vi "Test Sequence.vi"(0 "FeedBack Channel":string[](array[string])=["fgdgfvcbc", "vnfhgjkn", "21354682"], 1 "Test Name":string, 2 "Steps":T1(array[cluster]), 3 "Load":refnum<vi>, 4 "Lvdt":refnum<vi>) -> (6 "Emergency":bool, 7 "Out":i32, 8 "Condition":bool)   [LabVIEW 2020]
uses:
  Galobal variable_TI.vi
  Project Setup/Globle Variable/GR_Servo.vi
panel:
  out "Wait/Poll (ms)":u32
  out "Channels (Out)":i32[](array[numeric])
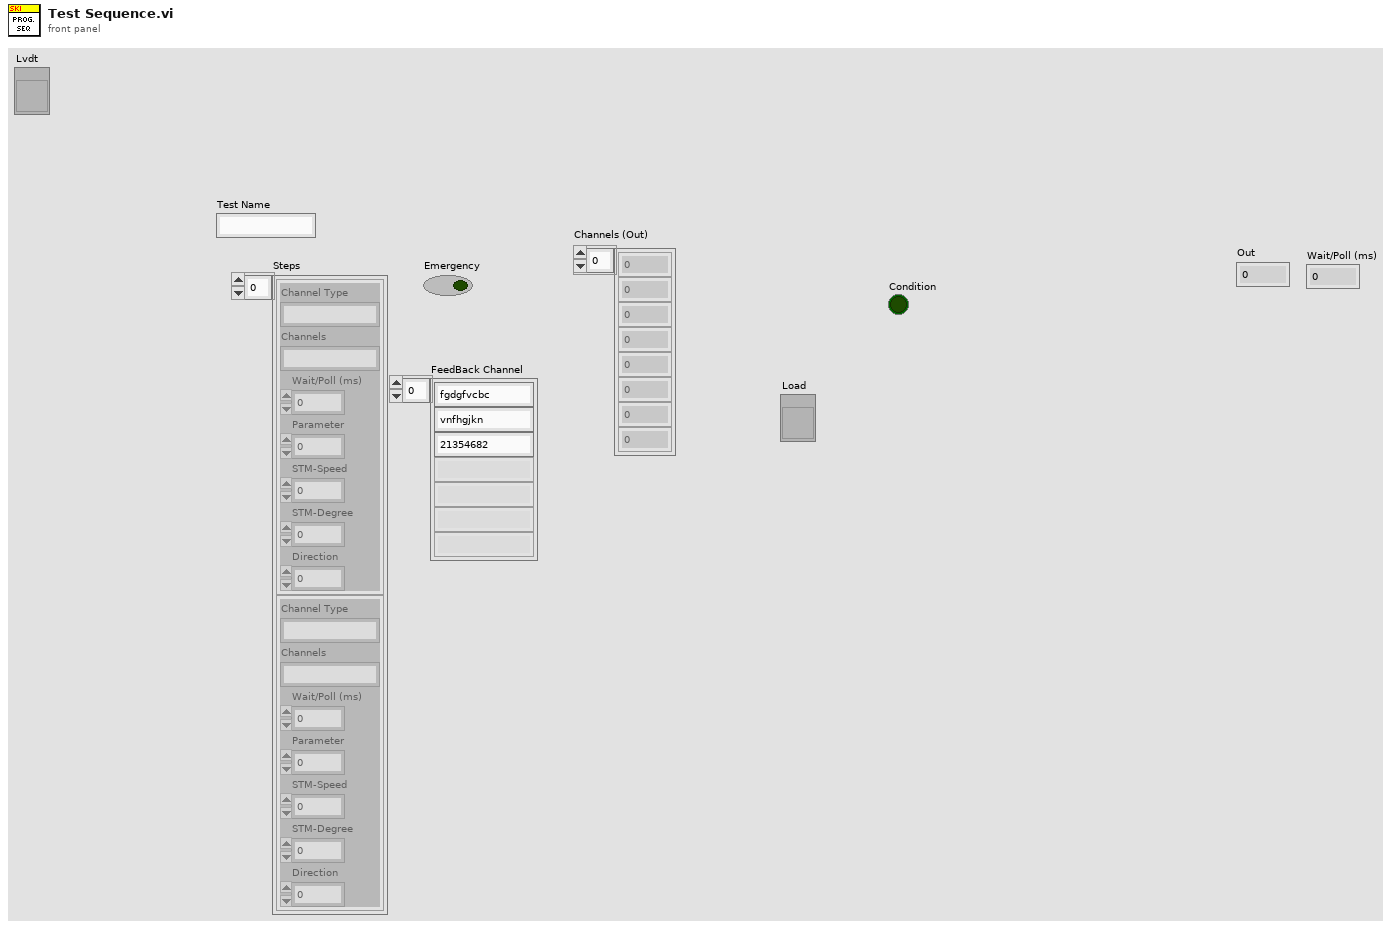
[diagram p1: front panel]
types:
  T1 = cluster{"Channel Type":string, "Channels":string, "Wait/Poll (ms)":u32, "Parameter":u8, "STM-Speed":i32, "STM-Degree":u32, "Direction":u8}[]
  T2 = cluster{"Emergency_1":bool, "Reset_2":bool, "Air Pressure_4":bool, "Safety Sensor_5":bool, "Safety Sensor_6":bool, "Barcode Rev rs_24":bool, "Clamp fwd rs_21":bool, "Servo Fault":bool, "Home _3":bool}
  T3 = cluster{"Start":bool, "Emergency ":bool, "Reset":bool, "Home":bool, "Safety":bool}
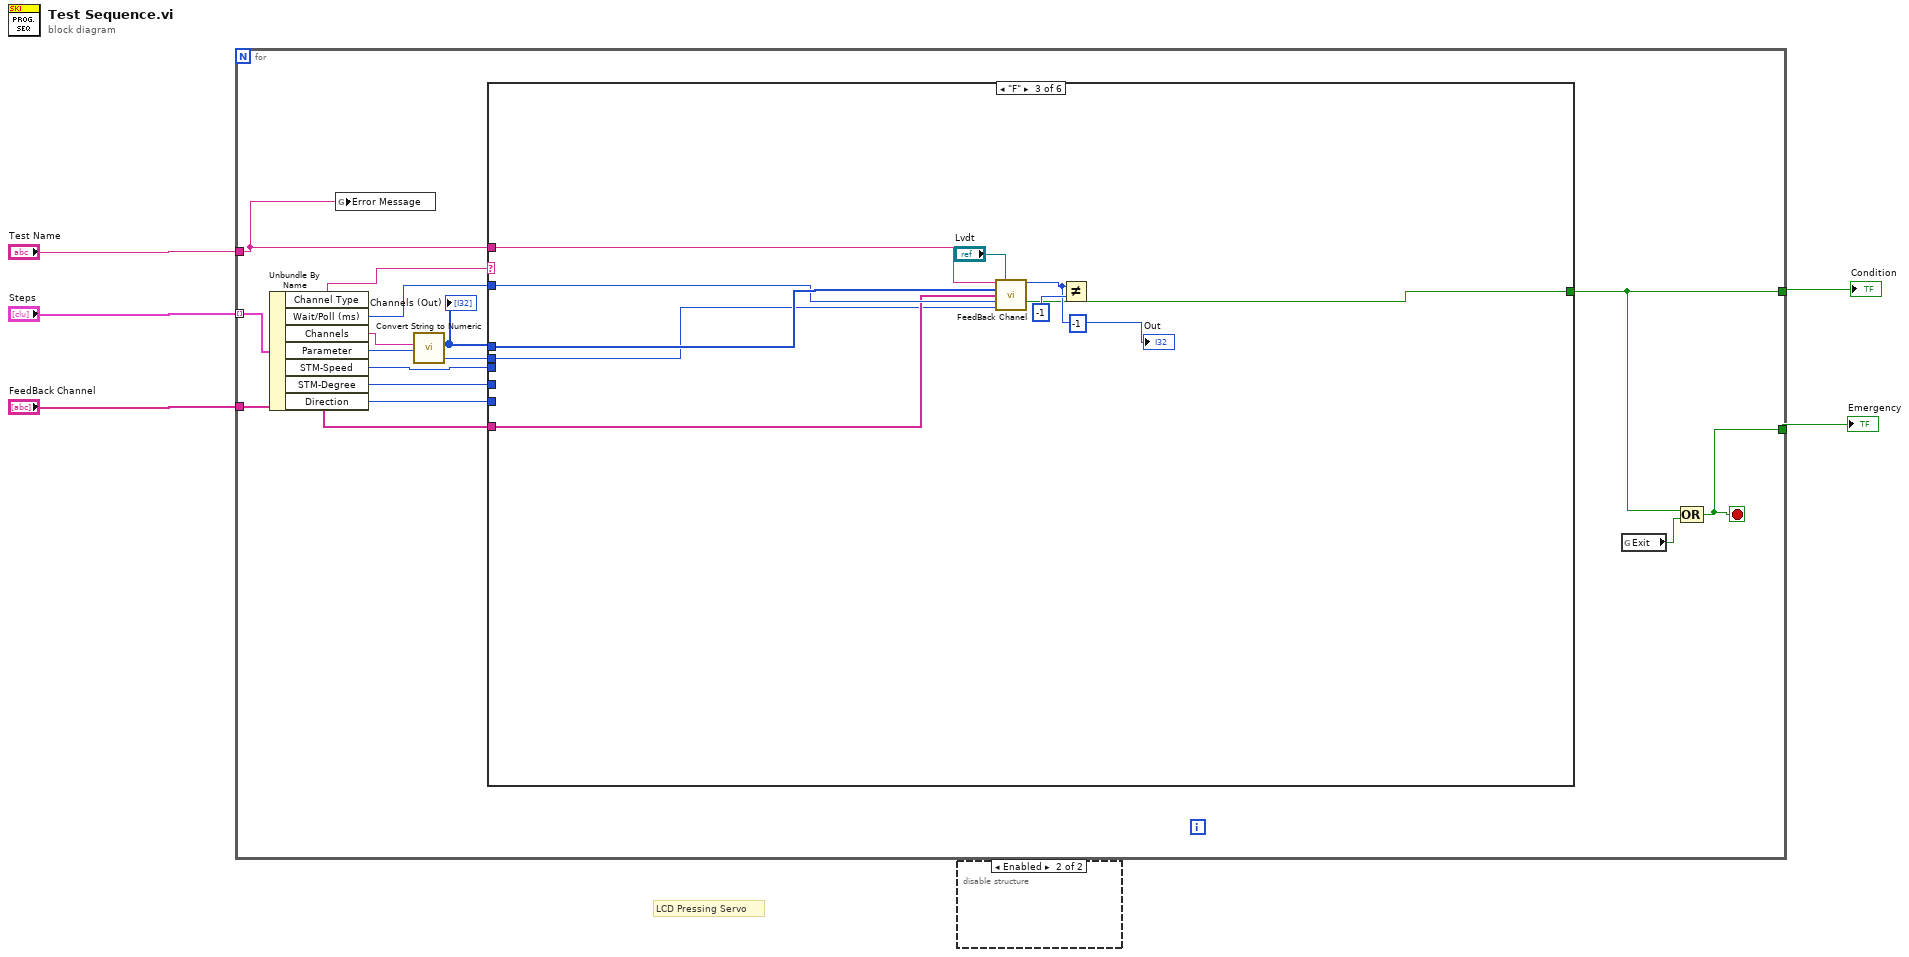
[diagram p0: block diagram]
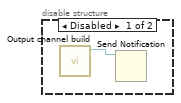
[diagram p2: hidden frame]
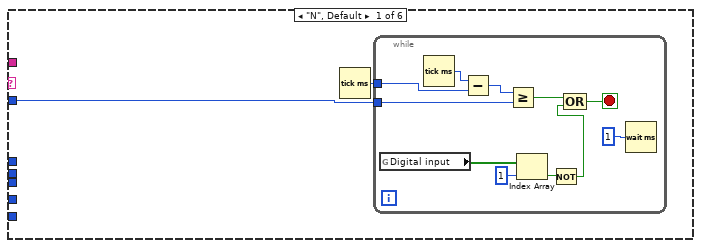
[diagram p3: hidden frame]
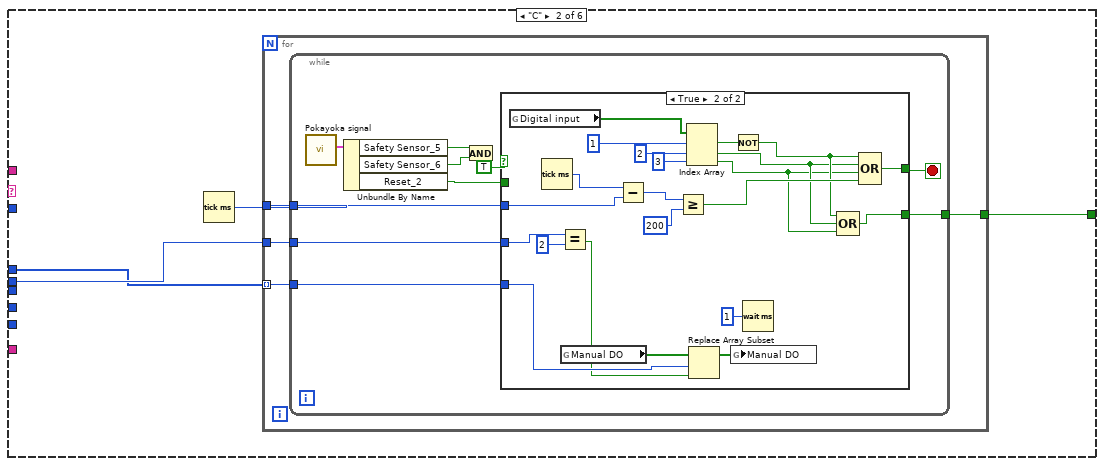
[diagram p4: hidden frame]
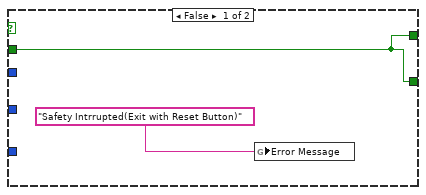
[diagram p5: hidden frame]
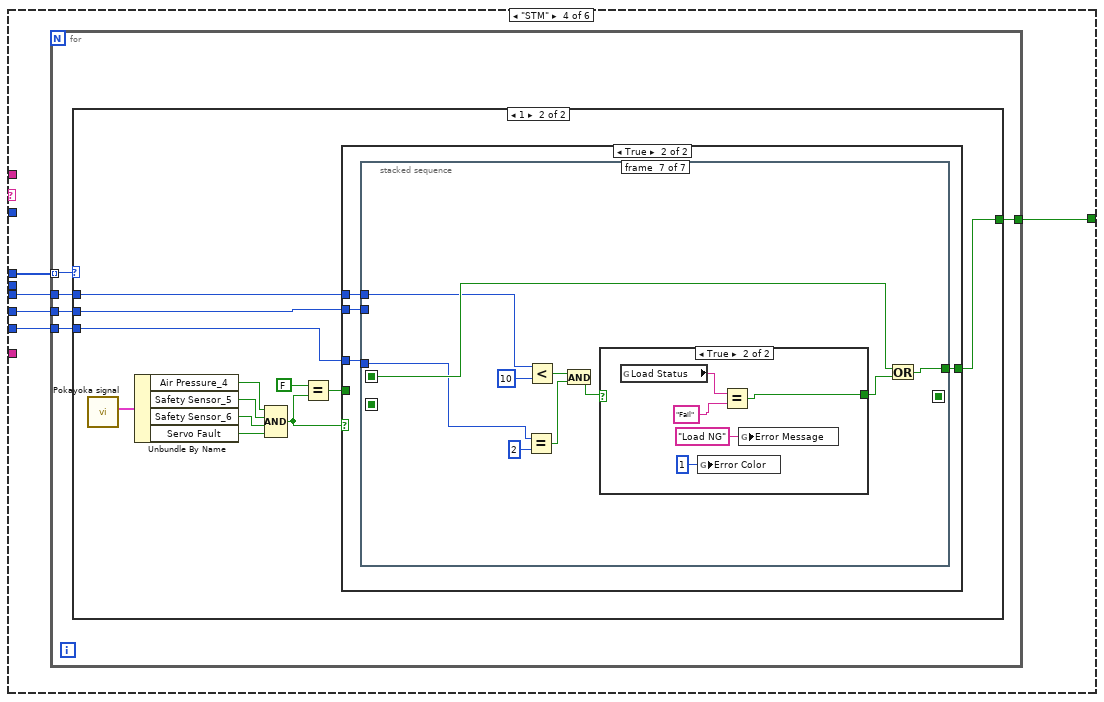
[diagram p6: hidden frame]
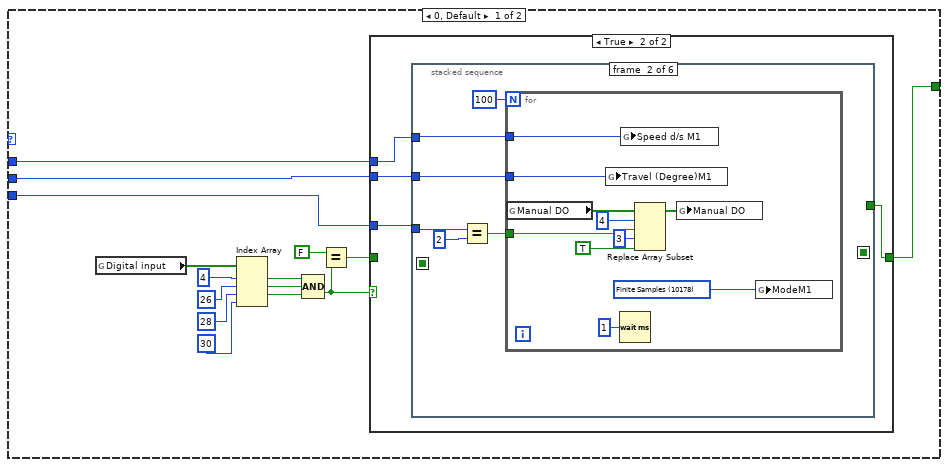
[diagram p7: hidden frame]
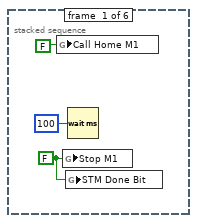
[diagram p9: hidden frame]
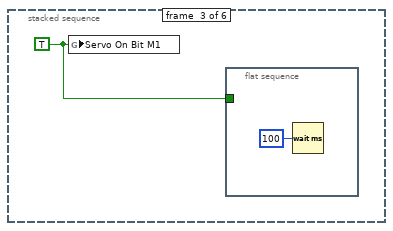
[diagram p10: hidden frame]
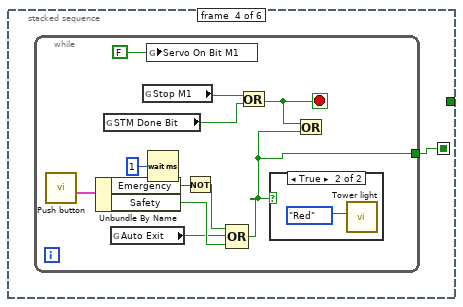
[diagram p11: hidden frame]
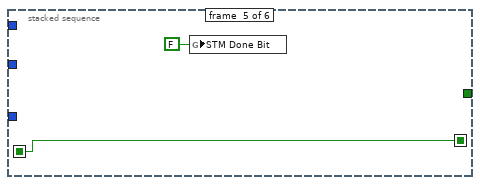
[diagram p13: hidden frame]
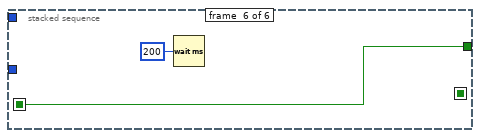
[diagram p14: hidden frame]
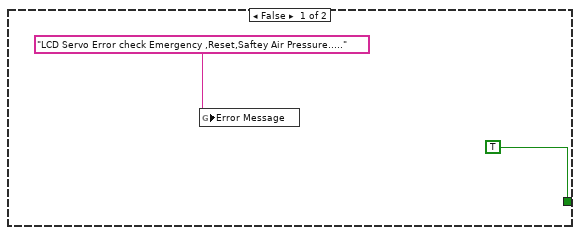
[diagram p15: hidden frame]
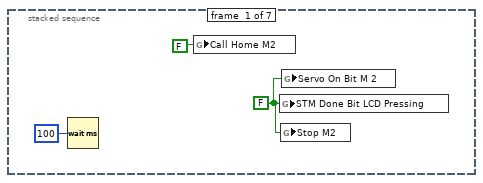
[diagram p16: hidden frame]
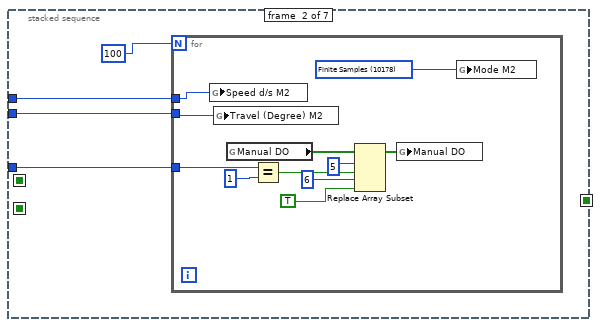
[diagram p17: hidden frame]
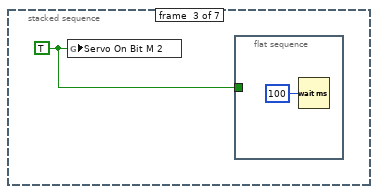
[diagram p18: hidden frame]
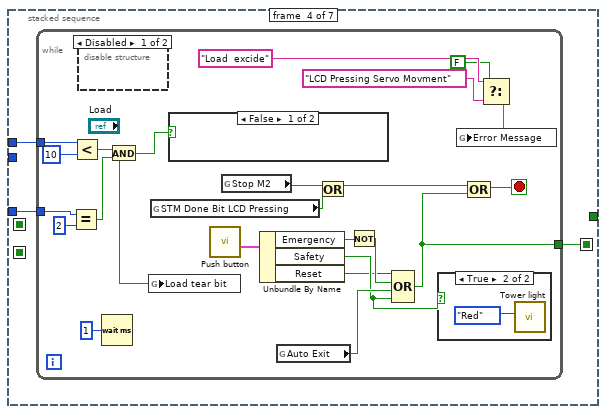
[diagram p19: hidden frame]
diagram:
  # "LCD Pressing Servo"
  n1 = for {
    tunnel: "Steps" -> [w19] mode=indexing
    tunnel: [w7] -> w5
    tunnel: "Test Name" -> [w6]
    tunnel: "FeedBack Channel" -> [w14]
    tunnel: [w12] -> w1
    stop <- w7 stop-if-true
    n2 = Unbundle By Name(w19) -> ("Channel Type"=w18:string, "Wait/Poll (ms)"=w17:u32, "Channels"=w16:string, "Parameter"=w8:u8, "STM-Speed"=w10:i32, "STM-Degree"=w9:u32, "Direction"=w11:u8)
    n3 = global write "GR_Servo.vi" "Error Message"(w6) -> ()
    n4 = call "Convert String to Numeric.vi"("Channels (A:B:C:D...) (In)"=w16) -> ("Channels (Out)"=w15:i32[])  [unwired: 9 in, 1 out]
    "Channels (Out)" <- w15
    n5 = case shown="\"F\"" w18 {
      tunnel: w17 -> [w20 _ w82 _ _ w277]
      tunnel: w15 -> [_ w34 w83 w88 w245 _]
      tunnel: w11 -> [_ _ _ w87 _ _]
      tunnel: w6 -> [_ _ w81 _ _ _]
      tunnel: w14 -> [_ _ w80 _ _ _]
      tunnel: [_ w33 w76 w84 w243 w273] -> w12
      tunnel: w10 -> [_ _ _ w86 _ _]
      tunnel: w9 -> [_ _ _ w85 _ _]
      tunnel: w8 -> [_ w36 w77 _ w244 w280]
      frame "N", Default {
        n6 = Tick Count (ms)() -> (millisecond timer value=w21:u32)
        n7 = while {
          tunnel: w21 -> [w31]
          tunnel: w20 -> [w26]
          stop <- w27 stop-if-true
          n8 = global read "Galobal variable_TI.vi" "Digital input"() -> (w25:bool[])
          n9 = Tick Count (ms)() -> (millisecond timer value=w32:u32)
          n10 = Subtract(x=w32, y=w31) -> (x-y=w30:u32)
          n11 = Greater Or Equal?(x=w30, y=w26) -> (x >= y?=w28:bool)
          n12 = Index Array(array=w25, index=1) -> (element=w23:bool)
          n13 = Not(x=w23) -> (.not. x?=w22:bool)
          n14 = Compound Arithmetic op=OR(w28, w22) -> (w27:bool)
          n15 = Wait (ms)(milliseconds to wait=u32 1) -> ()  [unwired: 1 out]
        }
      }
      frame "C" {
        n16 = Tick Count (ms)() -> (millisecond timer value=w35:u32)
        n17 = for {
          tunnel: w34 -> [w39] mode=indexing
          tunnel: w36 -> [w40]
          tunnel: w35 -> [w38]
          tunnel: [w37] -> w33
          n18 = while {
            tunnel: w40 -> [w50]
            tunnel: w39 -> [w49]
            tunnel: w38 -> [w48]
            tunnel: [w42] -> w37
            stop <- w43 stop-if-true
            n19 = call "Pokayoka signal.vi"() -> ("output cluster"=w47:T2)  [unwired: 10 in, 1 out]
            n20 = Unbundle By Name(w47) -> ("Safety Sensor_5"=w46:bool, "Safety Sensor_6"=w45:bool, "Reset_2"=w44:bool)
            n21 = And(x=w46, y=w45) -> ()  [unwired: 1 out]
            n22 = case shown="True" TRUE {
              tunnel: w50 -> [_ w74]
              tunnel: w49 -> [_ w73]
              tunnel: w48 -> [_ w72]
              tunnel: [w51 w71] -> w43
              tunnel: w44 -> [w51 _]
              tunnel: [w51 w53] -> w42
              frame False {
                n23 = global write "GR_Servo.vi" "Error Message"("Safety Intrrupted(Exit with Reset Button)") -> ()
              }
              frame True {
                n24 = global read "Galobal variable_TI.vi" "Digital input"() -> (w61:bool[])
                n25 = Tick Count (ms)() -> (millisecond timer value=w65:u32)
                n26 = Equal?(x=w74, y=u8 2) -> (x = y?=w66:bool)
                n27 = global read "Galobal variable_TI.vi" "Manual DO"() -> (w67:bool[])
                n28 = Subtract(x=w65, y=w72) -> (x-y=w64:u32)
                n29 = Greater Or Equal?(x=w64, y=u32 200) -> (x >= y?=w62:bool)
                n30 = Index Array(array=w61, index #1=1 ("index"), index #2=2 ("index"), index #3=3 ("index")) -> (element #1=w57:bool, element #2=w55:bool, element #3=w54:bool)
                n31 = Replace Array Subset(array=w67, new element=w66, index=w73) -> (w68:bool[])
                n32 = global write "Galobal variable_TI.vi" "Manual DO"(w68) -> ()
                n33 = Not(x=w57) -> (.not. x?=w56:bool)
                n34 = Wait (ms)(milliseconds to wait=u32 1) -> ()  [unwired: 1 out]
                n35 = Compound Arithmetic op=OR(w56, w55, w54) -> (w53:bool)
                n36 = Compound Arithmetic op=OR(w56, w55, w54, w62) -> (w71:bool)
              }
            }
          }
        }
      }
      frame "F" {
        (unwired) -1 ("Out")
        n37 = call "FeedBack Chanel.vi"("Test Name"=w81, "Lvdt"="Lvdt", "Channels (Int)"=w83, "FeedBack Channel"=w80, "Wait/Poll (ms)"=w82, "Parameter"=w77) -> ("Out"=w78:i32, "Fail"=w76:bool)  [unwired: 5 in, 3 out]
        "Out" <- w78
        n38 = Not Equal?(x=w78, y=-1) -> ()  [unwired: 1 out]
      }
      frame "STM" {
        n39 = for {
          tunnel: w88 -> [w93] mode=indexing
          tunnel: w87 -> [w92]
          tunnel: w86 -> [w91]
          tunnel: w85 -> [w90]
          tunnel: [w89] -> w84
          n40 = case shown="1" w93 {
            tunnel: w92 -> [w106 w159]
            tunnel: w91 -> [w108 w161]
            tunnel: w90 -> [w107 w160]
            tunnel: [w94 w158] -> w89
            frame 0, Default {
              n41 = global read "Galobal variable_TI.vi" "Digital input"() -> (w98:bool[])
              n42 = Index Array(array=w98, index #1=4 ("index"), index #2=26 ("index"), index #3=28 ("index"), index #4=30 ("index")) -> (element #1=w105:bool, element #2=w102:bool, element #3=w103:bool)  [unwired: 1 out]
              n43 = Compound Arithmetic op=AND(w105, w102, w103) -> (w97:bool)
              n44 = Equal?(x=FALSE ("y"), y=w97) -> (x = y?=w95:bool)
              n45 = case shown="True" w97 {
                tunnel: w108 -> [_ w113]
                tunnel: w107 -> [_ w112]
                tunnel: w106 -> [_ w111]
                tunnel: [w109 w110] -> w94
                tunnel: w95 -> [w109 _]
                frame False {
                }
                frame True {
                  n46 = stacked-sequence {
                    seq-local: [_ _ _ w135 _ _] -> [_ _ _ _ w148 _]
                    seq-local: [_ _ _ _ w148 _] -> [_ _ _ _ _ w150]
                    tunnel: w112 -> [_ w122 _ _ _ _]
                    tunnel: w111 -> [_ w120 _ _ _ _]
                    tunnel: w113 -> [_ w118 _ _ _ _]
                    tunnel: [_ _ _ _ _ w150] -> w110
                    frame #0 {
                      w114 = FALSE ("Stop M1")
                      n47 = global write "Galobal variable_TI.vi" "Call Home M1"(FALSE ("Call Home M2")) -> ()
                      n48 = global write "Galobal variable_TI.vi" "Stop M1"(w114) -> ()
                      n49 = global write "Galobal variable_TI.vi" "STM Done Bit"(w114) -> ()
                      n50 = Wait (ms)(milliseconds to wait=u32 100) -> ()  [unwired: 1 out]
                    }
                    frame #1 {
                      n51 = Equal?(x=w120, y=u8 2) -> (x = y?=w119:bool)
                      n52 = for {
                        N: 100 -> [_]
                        tunnel: w122 -> [w132]
                        tunnel: w119 -> [w130]
                        tunnel: w118 -> [w128]
                        w131 = 10178 items=["Finite Samples"=10178, "Continuous Samples"=10123, "Hardware Timed Single Point"=12522] ("ModeM1")
                        n53 = global read "Galobal variable_TI.vi" "Manual DO"() -> (w126:bool[])
                        n54 = global write "GR_Servo.vi" "Travel (Degree)M1"(w132) -> ()
                        n55 = Wait (ms)(milliseconds to wait=u32 1) -> ()  [unwired: 1 out]
                        n56 = global write "GR_Servo.vi" "Speed d/s M1"(w128) -> ()
                        n57 = Replace Array Subset(array=w126, new element #1=w130, index #1=4 ("index"), new element #2=TRUE ("new element/subarray"), index #2=3 ("index")) -> (w129:bool[])
                        n58 = global write "Galobal variable_TI.vi" "Manual DO"(w129) -> ()
                        n59 = global write "GR_Servo.vi" "ModeM1"(w131) -> ()
                      }
                    }
                    frame #2 {
                      w133 = TRUE ("Servo On Bit")
                      n60 = global write "GR_Servo.vi" "Servo On Bit M1"(w133) -> ()
                      n61 = flat-sequence {
                        tunnel: w133 -> [_]
                        frame #0 {
                          n62 = Wait (ms)(milliseconds to wait=u32 100) -> ()  [unwired: 1 out]
                        }
                      }
                    }
                    frame #3 {
                      n63 = while {
                        tunnel: [w136] -> w135
                        stop <- w142 stop-if-true
                        n64 = call "Push button.vi"() -> ("Push Button"=w137:T3)  [unwired: 11 in]
                        n65 = Unbundle By Name(w137) -> ("Emergency"=w138:bool, "Safety"=w141:bool)
                        n66 = global read "Galobal variable_TI.vi" "STM Done Bit"() -> (w144:bool)
                        n67 = global read "Galobal variable_TI.vi" "Auto Exit"() -> (w139:bool)
                        n68 = global read "Galobal variable_TI.vi" "Stop M1"() -> (w145:bool)
                        n69 = global write "GR_Servo.vi" "Servo On Bit M1"(FALSE ("Servo On Bit")) -> ()
                        n70 = Wait (ms)(milliseconds to wait=u32 1) -> ()  [unwired: 1 out]
                        n71 = Not(x=w138) -> (.not. x?=w140:bool)
                        n72 = Compound Arithmetic op=OR(w140, w139, w141) -> (w136:bool)
                        n73 = Or(x=w145, y=w144) -> (x .or. y?=w142:bool)
                        n74 = case shown="True" w136 {
                          frame False {
                          }
                          frame True {
                            n75 = call "Tower light.vi"("Enum"=enum16{"Green", "Red", "Yellow", "OFF"}."Red") -> ()  [unwired: 11 in]
                          }
                        }
                        n76 = Or(x=w142, y=w136) -> ()  [unwired: 1 out]
                      }
                    }
                    frame #4 {
                      n77 = global write "Galobal variable_TI.vi" "STM Done Bit"(FALSE ("STM Done Bit LCD Pressing")) -> ()
                    }
                    frame #5 {
                      n78 = Wait (ms)(milliseconds to wait=u32 200) -> ()  [unwired: 1 out]
                    }
                  }
                }
              }
            }
            frame 1 {
              n79 = call "Pokayoka signal.vi"() -> ("output cluster"=w157:T2)  [unwired: 10 in, 1 out]
              n80 = Unbundle By Name(w157) -> ("Air Pressure_4"=w156:bool, "Safety Sensor_5"=w155:bool, "Safety Sensor_6"=w154:bool, "Servo Fault"=w152:bool)
              n81 = Compound Arithmetic op=AND(w156, w155, w154, w152) -> (w153:bool)
              n82 = Equal?(x=FALSE ("y"), y=w153) -> (x = y?=w162:bool)
              n83 = case shown="True" w153 {
                tunnel: w161 -> [_ w169]
                tunnel: w160 -> [_ w168]
                tunnel: w159 -> [_ w167]
                tunnel: w162 -> [_ _]
                tunnel: [TRUE w166] -> w158
                frame False {
                  n84 = global write "GR_Servo.vi" "Error Message"("LCD Servo Error check Emergency ,Reset,Saftey Air Pressure.....") -> ()
                }
                frame True {
                  n85 = stacked-sequence {
                    seq-local: [_ _ _ w192 _ _ _] -> [_ _ _ _ w217 _ _]
                    seq-local: [_ _ _ _ w217 _ _] -> [_ _ _ _ _ w222 _]
                    seq-local: [_ _ _ _ _ w222 _] -> [_ _ _ _ _ _ w236]
                    tunnel: w168 -> [_ w176 _ _ _ _ _]
                    tunnel: w167 -> [_ w175 _ w191 _ _ w228]
                    tunnel: w169 -> [_ w174 _ w190 _ _ w229]
                    tunnel: [_ _ _ _ _ _ w234] -> w166
                    frame #0 {
                      w170 = FALSE ("STM Done Bit LCD Pressing")
                      n86 = Wait (ms)(milliseconds to wait=u32 100) -> ()  [unwired: 1 out]
                      n87 = global write "Galobal variable_TI.vi" "Call Home M2"(FALSE ("Call Home M2")) -> ()
                      n88 = global write "GR_Servo.vi" "STM Done Bit LCD Pressing"(w170) -> ()
                      n89 = global write "Galobal variable_TI.vi" "Stop M2"(w170) -> ()
                      n90 = global write "GR_Servo.vi" "Servo On Bit M 2"(w170) -> ()
                    }
                    frame #1 {
                      n91 = for {
                        N: 100 -> [_]
                        tunnel: w176 -> [w187]
                        tunnel: w175 -> [w184]
                        tunnel: w174 -> [w181]
                        w186 = 10178 items=["Finite Samples"=10178, "Continuous Samples"=10123, "Hardware Timed Single Point"=12522] ("ModeM1")
                        n92 = global write "GR_Servo.vi" "Speed d/s M2"(w181) -> ()
                        n93 = global write "GR_Servo.vi" "Travel (Degree) M2"(w187) -> ()
                        n94 = global read "Galobal variable_TI.vi" "Manual DO"() -> (w179:bool[])
                        n95 = Equal?(x=w184, y=u8 1) -> (x = y?=w183:bool)
                        n96 = Replace Array Subset(array=w179, new element #1=w183, index #1=5 ("index"), new element #2=TRUE ("new element/subarray"), index #2=6 ("index")) -> (w182:bool[])
                        n97 = global write "Galobal variable_TI.vi" "Manual DO"(w182) -> ()
                        n98 = global write "GR_Servo.vi" "Mode M2"(w186) -> ()
                      }
                    }
                    frame #2 {
                      w188 = TRUE ("Servo On Bit")
                      n99 = global write "GR_Servo.vi" "Servo On Bit M 2"(w188) -> ()
                      n100 = flat-sequence {
                        tunnel: w188 -> [_]
                        frame #0 {
                          n101 = Wait (ms)(milliseconds to wait=u32 100) -> ()  [unwired: 1 out]
                        }
                      }
                    }
                    frame #3 {
                      n102 = while {
                        tunnel: [w206] -> w192
                        tunnel: w191 -> [w201]
                        tunnel: w190 -> [w199]
                        stop <- w207 stop-if-true
                        n103 = Equal?(x=w201, y=u8 2) -> (x = y?=w196:bool)
                        n104 = Less?(x=w199, y=10) -> (x < y?=w197:bool)
                        n105 = disable-structure shown="Disabled" {
                          frame Disabled {
                          }
                          frame Enabled {
                          }
                        }
                        n106 = Wait (ms)(milliseconds to wait=u32 1) -> ()  [unwired: 1 out]
                        n107 = And(x=w197, y=w196) -> (x .and. y?=w194:bool)
                        n108 = global write "Galobal variable_TI.vi" "Load tear bit"(w194) -> ()
                        n109 = global read "GR_Servo.vi" "STM Done Bit LCD Pressing"() -> (w213:bool)
                        n110 = case shown="False" w194 {
                          frame False {
                          }
                          frame True {
                          }
                        }
                        n111 = call "Push button.vi"() -> ("Push Button"=w212:T3)  [unwired: 11 in]
                        n112 = global read "Galobal variable_TI.vi" "Stop M2"() -> (w214:bool)
                        n113 = Unbundle By Name(w212) -> ("Emergency"=w211:bool, "Safety"=w205:bool, "Reset"=w193:bool)
                        n114 = global read "Galobal variable_TI.vi" "Auto Exit"() -> (w210:bool)
                        n115 = Or(x=w214, y=w213) -> (x .or. y?=w208:bool)
                        n116 = Not(x=w211) -> (.not. x?=w209:bool)
                        n117 = Compound Arithmetic op=OR(w193, w209, w210, w205) -> (w206:bool)
                        n118 = case shown="True" w205 {
                          frame False {
                          }
                          frame True {
                            n119 = call "Tower light.vi"("Enum"=enum16{"Green", "Red", "Yellow", "OFF"}."Red") -> ()  [unwired: 11 in]
                          }
                        }
                        n120 = Compound Arithmetic op=OR(w208, w206) -> (w207:bool)
                        n121 = Select(t="Load  excide", s=FALSE, f="LCD Pressing Servo Movment") -> (s? t:f=w202:string)
                        n122 = global write "GR_Servo.vi" "Error Message"(w202) -> ()
                      }
                    }
                    frame #4 {
                      (unwired) FALSE
                      n123 = Wait (ms)(milliseconds to wait=u32 1) -> ()  [unwired: 1 out]
                      n124 = global write "GR_Servo.vi" "Servo On Bit M 2"(FALSE ("Servo On Bit")) -> ()
                      n125 = global write "GR_Servo.vi" "STM Done Bit LCD Pressing"(FALSE ("STM Done Bit LCD Pressing")) -> ()
                    }
                    frame #5 {
                      n126 = disable-structure shown="Disabled" {
                        frame Disabled {
                          n127 = local read "Load"() -> (w224:refnum<vi>)
                          n128 = call "Load Value.vi"("String in"=w224) -> (1:w225, "Load Cell"=w226:dbl)  [unwired: 9 in]
                          n129 = Greater?(x=w226, y=w225) -> ()  [unwired: 1 out]
                        }
                        frame Enabled {
                        }
                      }
                      n130 = Wait (ms)(milliseconds to wait=u32 100) -> ()  [unwired: 1 out]
                      n131 = global write "Galobal variable_TI.vi" "Load tear bit"(FALSE ("Load tear bit")) -> ()
                    }
                    frame #6 {
                      n132 = Equal?(x=w228, y=u8 2) -> (x = y?=w233:bool)
                      n133 = Less?(x=w229, y=10) -> (x < y?=w232:bool)
                      n134 = And(x=w232, y=w233) -> (x .and. y?=w227:bool)
                      n135 = case shown="True" w227 {
                        tunnel: [FALSE w240] -> w235
                        frame False {
                        }
                        frame True {
                          n136 = global read "Galobal variable_TI.vi" "Load Status"() -> (w241:string)
                          n137 = global write "GR_Servo.vi" "Error Color"(1 ("Error Color")) -> ()
                          n138 = Equal?(x=w241, y="Fail") -> (x = y?=w240:bool)
                          n139 = global write "GR_Servo.vi" "Error Message"("Load NG" ("Error Message")) -> ()
                        }
                      }
                      n140 = Or(x=w236, y=w235) -> (x .or. y?=w234:bool)
                    }
                  }
                }
              }
            }
          }
        }
      }
      frame "CAM" {
        n141 = for {
          tunnel: w245 -> [w248] mode=indexing
          tunnel: w244 -> [w247]
          tunnel: [w246] -> w243
          n142 = case shown="0, Default" w248 {
            tunnel: w247 -> [_ _]
            tunnel: [w249 _] -> w246
            frame 0, Default {
              n143 = stacked-sequence {
                seq-local: [_ w251 _] -> [_ _ w269]
                tunnel: [_ _ w269] -> w249
                frame #0 {
                  n144 = global write "Galobal variable_TI.vi" "CAM Trigger"(TRUE ("CAM Trigger")) -> ()
                }
                frame #1 {
                  n145 = while {
                    tunnel: [w261] -> w251
                    i -> [w256]
                    stop <- w263 stop-if-true
                    n146 = global read "Galobal variable_TI.vi" "Digital input"() -> (w260:bool[])
                    n147 = Greater?(x=w256, y=6000) -> (0:w254:bool)
                    n148 = call "Push button.vi"() -> ("Push Button"=w267:T3)  [unwired: 11 in]
                    n149 = global read "Galobal variable_TI.vi" "ok"() -> (w253:bool)
                    n150 = Unbundle By Name(w267) -> ("Emergency"=w266:bool, "Reset"=w264:bool)
                    n151 = Index Array(array=w260, index #1=12 ("index"), index #2=13 ("index")) -> ()  [unwired: 2 out]
                    n152 = global read "Galobal variable_TI.vi" "ng"() -> (w252:bool)
                    n153 = Not(x=w266) -> (.not. x?=w265:bool)
                    n154 = Compound Arithmetic op=OR(w265, w264, w252, w252, w254) -> (w261:bool)
                    n155 = global write "GR_Servo.vi" "Error Message"("Waitting for camera......" ("Error Message")) -> ()
                    n156 = Wait (ms)(milliseconds to wait=u32 1) -> ()  [unwired: 1 out]
                    n157 = Compound Arithmetic op=OR(w261, w253, w253) -> (w263:bool)
                  }
                }
                frame #2 {
                  n158 = global write "Galobal variable_TI.vi" "Camera Result"("" ("Camera Result")) -> ()
                  n159 = global write "Galobal variable_TI.vi" "CAM Trigger"(FALSE ("CAM Trigger")) -> ()
                }
              }
            }
            frame 1 {
              # "LCD Pressing Servo"
            }
          }
        }
      }
      frame "BAR" {
        n160 = Equal?(x=w280, y=u8 2) -> (x = y?=w278:bool)
        n161 = case shown="1" w277 {
          tunnel: w278 -> [w289 w297]
          tunnel: [w291 w296] -> w272
          tunnel: [w290 _] -> _
          tunnel: [FALSE TRUE] -> w271
          frame 1 {
            n162 = case shown="True" w289 {
              tunnel: [FALSE ("exit") w294] -> w291
              tunnel: [_ TRUE] -> w290
              frame False {
              }
              frame True {
                n163 = call "Barcode read.vi"() -> ("exit"=w294:bool)  [unwired: 8 in, 3 out]
              }
            }
          }
          frame 0, Default {
            n164 = case shown="True" w297 {
              tunnel: [FALSE ("exit") w299] -> w296
              frame False {
              }
              frame True {
                n165 = call "TFT_Barcode read.vi"() -> ("exit"=w299:bool)  [unwired: 8 in, 3 out]
              }
            }
          }
        }
        n166 = global read "Galobal variable_TI.vi" "Tracibility"() -> (w276:bool)
        n167 = And(x=w271, y=w276) -> (x .and. y?=w275:bool)
        n168 = case shown="False" w275 {
          tunnel: [FALSE ("Fail") w283] -> w274
          frame False {
            n169 = global write "Galobal variable_TI.vi" "Rework bit"(TRUE ("Rework bit")) -> ()
          }
          frame True {
            n170 = flat-sequence {
              tunnel: [w286] -> w283
              frame #0 {
                n171 = global write "Galobal variable_TI.vi" "Rpt Read"(TRUE ("Rpt Read")) -> ()
              }
              frame #1 {
                n172 = Wait (ms)(milliseconds to wait=u32 500) -> ()  [unwired: 1 out]
              }
              frame #2 {
                n173 = call "RPT Comaristion.vi"("True"=TRUE) -> ("Fail"=w286:bool)  [unwired: 10 in]
              }
            }
          }
        }
        n174 = Or(x=w272, y=w274) -> (x .or. y?=w273:bool)
        "Wait/Poll (ms)" <- w277
      }
    }
    n175 = global read "Galobal variable_TI.vi" "Exit"() -> (w13:bool)
    n176 = Compound Arithmetic op=OR(w12, w13) -> (w7:bool)
  }
  "Emergency" <- w5
  "Condition" <- w1
  n177 = disable-structure shown="Enabled" {
    frame Disabled {
      n178 = call "Output channel build.vi"() -> ("Output channel"=w300:refnum<notifier>)  [unwired: 11 in]
      n179 = Send Notification(notifier=w300) -> ()  [unwired: 2 in, 2 out]
    }
    frame Enabled {
    }
  }
